vi "CB Flywheel.vi"(5 "moment of intertia":dbl, 6 "encoder?":bool=TRUE, 7 "gear ratio":dbl, 8 "dt":dbl=-1.0, 10 "num motors":i32=1, 11 "Motor ID":T3) -> (3 "Discrete SSM":T1)   [LabVIEW 2020]
uses:
  Motors/CB Motor ID.ctl
  CB State Space.ctl
  <vilib>/Analysis/Matrix/Datatypes/RealMatrix.ctl
  <vilib>/Analysis/Matrix/NI_Matrix.lvlib
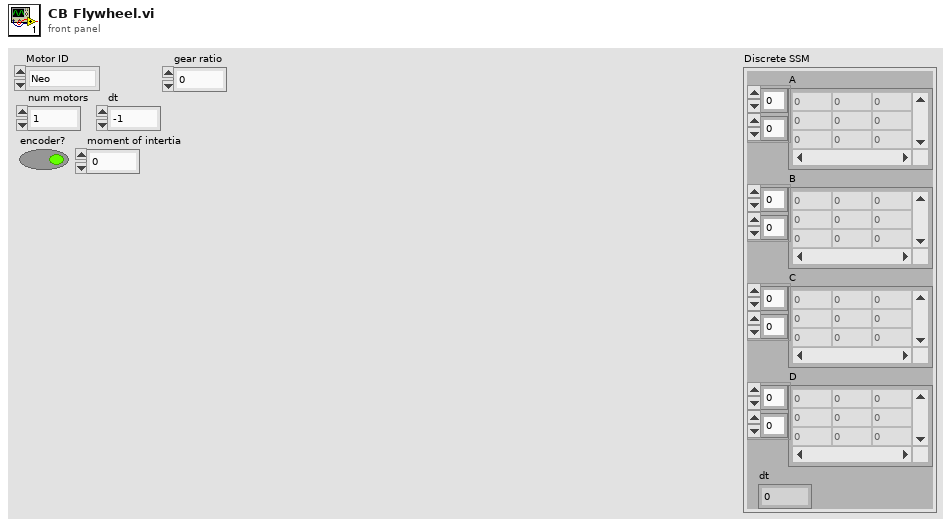
[diagram p1: front panel]
types:
  T1 = typedef "CB State Space.ctl" = cluster{"A":T2, "B":T2, "C":T2, "D":T2, "dt":dbl}
  T2 = typedef "NI_Matrix.lvlib/RealMatrix.ctl" = dbl[][]
  T3 = typedef "CB Motor ID.ctl" = enum16{"Neo", "Neo 550", "Falcon 500", "775pro"}
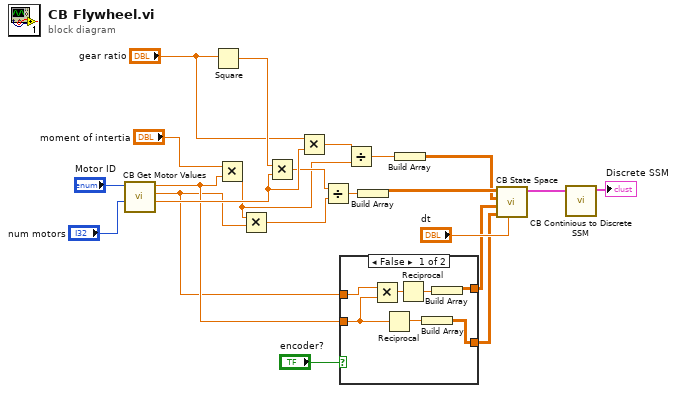
[diagram p0: block diagram]
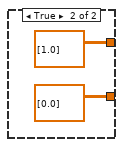
[diagram p2: hidden frame]
diagram:
  n1 = call "CB Get Motor Values.vi"("num motors"="num motors", "Motor ID"="Motor ID") -> ("Kt"=w13:dbl, "Kv"=w1:dbl, "R"=w2:dbl)  [unwired: 6 in, 1 out]
  n2 = Square(x="gear ratio") -> (x^2=w14:dbl)
  n3 = Multiply(x="moment of intertia", y=w2) -> (x*y=w7:dbl)
  n4 = Multiply(x=w7, y=w1) -> (x*y=w9:dbl)
  n5 = Multiply(x=w14, y=w13) -> (x*y=w10:dbl)
  n6 = Multiply(x="gear ratio", y=w13) -> (x*y=w8:dbl)
  n7 = Divide(x=w10, y=w9) -> (x/y=w6:dbl)
  n8 = case shown="False" "encoder?" {
    tunnel: [w23 T2 [[1.0]] ("C")] -> w17
    tunnel: [w28 T2 [[0.0]] ("D")] -> w16
    tunnel: w2 -> [w27 _]
    tunnel: w1 -> [w26 _]
    frame False {
      n9 = Multiply(x=w26, y=w27) -> (x*y=w25:dbl)
      n10 = Reciprocal(x=w27) -> (1/x=w29:dbl)
      n11 = Reciprocal(x=w25) -> (1/x=w24:dbl)
      n12 = Build Array(w29) -> (w28:T2)
      n13 = Build Array(w24) -> (w23:T2)
    }
    frame True {
    }
  }
  n14 = Divide(x=w8, y=w7) -> (x/y=w4:dbl)
  n15 = Build Array(w6) -> (w5:T2)
  n16 = Build Array(w4) -> (w3:T2)
  n17 = call "CB State Space.vi"("dt"="dt", "D"=w16, "C"=w17, "B"=w3, "A"=w5) -> ("State Space Model"=w19:T1)  [unwired: 5 in, 1 out]
  n18 = call "CB Continious to Discrete SSM.vi"("Cont SSM"=w19) -> ("Discrete SSM"=→"Discrete SSM":T1)  [unwired: 10 in]
